vi "GUI.Config Pulse generator.vi"(8 "error in":errorcluster, 10 "Config HW":T2={"VISA Rigol DP832"="FA_Rigol_DP832", "Config Rigol DP832"=[], "CTA Test#"="", "FT_Handle"=0, "Espera acceso FT"=0, "VISA Tek MDO3104"="Osciloscopio_Tek_MDO3104", "VISA Key 81160A"="Generator_Key_81160A"} {"Config Rigol DP832"."Channel" items=["+30V Channel 1", "+30V Channel 2", "+5V Channel 3"]; "Config Rigol DP832"."V Limit" format="%.1g"; "Config Rigol DP832"."I Limit" format="%.1g"; "Config Rigol DP832"."V Out" format="%.1g"}, 11 "CONFIG GEN origen":T1[](array[typedef]) {"Vasic Theorical" min=1.0 max=1000000.0 step=1.0 format="%#_6pV"; "Frequency" min=0.001 max=333000000.0 step=1000.0 format="%#_6pHz"; "Leading Edge Time" min=1e-09 max=1.0 step=1e-10 format="%#_6ps"; "Trailing Edge Time" min=1e-09 max=1.0 step=1e-10 format="%#_6ps"; "Delay" min=0.0 max=1.0 step=1e-12 format="%#_6ps"; "Trigger Level Sync" items=["ECL", "TTL"]; "Trigger Sync Out" items=["AB"=3, "B"=2, "A"=1, "None"=0]; "Load" min=1.0 max=1000000.0 step=1.0 format="%#_6p"; "DC Offset" min=-10.0 max=10.0 step=0.1 format="%#_6pV"; "Amplitude" min=0.05 max=5.0 step=0.001 format="%#_6pV"; "Width Time" min=1.5e-09 max=1.0 step=1e-10 format="%#_6ps"; "Channel" items=["Channel1"=1, "Channel2"=2]}) -> (0 "error out":errorcluster={"status"=TRUE, "code"=-1073807346, "source"="Property Node (arg 1) in DP832_Write.vi->DP832_Enable ALL Output.vi->GUI.Config Pulse generator.vi"}, 3 "Array pulse Out":T1[](array[typedef])=[{"Channel"=1, "Frequency"=1000000.0, "Width Time"=3.3e-09, "Amplitude"=0.05, "DC Offset"=0.0, "Load"=500.0, "Leading Edge Time"=1e-09, "Trailing Edge Time"=1e-09, "Delay"=0.0, "Out"=TRUE, "/Out"=TRUE, "Trigger Level Sync"=1, "Trigger Sync Out"=1, "Vasic Theorical"=50.0}, {"Channel"=1, "Frequency"=1000000.0, "Width Time"=3.3e-09, "Amplitude"=0.1, "DC Offset"=0.0, "Load"=500.0, "Leading Edge Time"=1e-09, "Trailing Edge Time"=1e-09, "Delay"=0.0, "Out"=TRUE, "/Out"=TRUE, "Trigger Level Sync"=1, "Trigger Sync Out"=1, "Vasic Theorical"=50.0}, {"Channel"=1, "Frequency"=1000000.0, "Width Time"=3.3e-09, "Amplitude"=0.2, "DC Offset"=0.0, "Load"=500.0, "Leading Edge Time"=1e-09, "Trailing Edge Time"=1e-09, "Delay"=0.0, "Out"=TRUE, "/Out"=TRUE, "Trigger Level Sync"=1, "Trigger Sync Out"=1, "Vasic Theorical"=50.0}, {"Channel"=1, "Frequency"=1000000.0, "Width Time"=3.3e-09, "Amplitude"=0.3, "DC Offset"=0.0, "Load"=500.0, "Leading Edge Time"=1e-09, "Trailing Edge Time"=1e-09, "Delay"=0.0, "Out"=TRUE, "/Out"=TRUE, "Trigger Level Sync"=1, "Trigger Sync Out"=1, "Vasic Theorical"=50.0}, {"Channel"=1, "Frequency"=1000000.0, "Width Time"=3.3e-09, "Amplitude"=0.4, "DC Offset"=0.0, "Load"=500.0, "Leading Edge Time"=1e-09, "Trailing Edge Time"=1e-09, "Delay"=0.0, "Out"=TRUE, "/Out"=TRUE, "Trigger Level Sync"=1, "Trigger Sync Out"=1, "Vasic Theorical"=50.0}, {"Channel"=1, "Frequency"=1000000.0, "Width Time"=3.3e-09, "Amplitude"=0.5, "DC Offset"=0.0, "Load"=500.0, "Leading Edge Time"=1e-09, "Trailing Edge Time"=1e-09, "Delay"=0.0, "Out"=TRUE, "/Out"=TRUE, "Trigger Level Sync"=1, "Trigger Sync Out"=1, "Vasic Theorical"=50.0}, {"Channel"=1, "Frequency"=1000000.0, "Width Time"=3.3e-09, "Amplitude"=0.6, "DC Offset"=0.0, "Load"=500.0, "Leading Edge Time"=1e-09, "Trailing Edge Time"=1e-09, "Delay"=0.0, "Out"=TRUE, "/Out"=TRUE, "Trigger Level Sync"=1, "Trigger Sync Out"=1, "Vasic Theorical"=50.0}, {"Channel"=1, "Frequency"=1000000.0, "Width Time"=3.3e-09, "Amplitude"=0.7, "DC Offset"=0.0, "Load"=500.0, "Leading Edge Time"=1e-09, "Trailing Edge Time"=1e-09, "Delay"=0.0, "Out"=TRUE, "/Out"=TRUE, "Trigger Level Sync"=1, "Trigger Sync Out"=1, "Vasic Theorical"=50.0}, {"Channel"=1, "Frequency"=1000000.0, "Width Time"=3.3e-09, "Amplitude"=0.8, "DC Offset"=0.0, "Load"=500.0, "Leading Edge Time"=1e-09, "Trailing Edge Time"=1e-09, "Delay"=0.0, "Out"=TRUE, "/Out"=TRUE, "Trigger Level Sync"=1, "Trigger Sync Out"=1, "Vasic Theorical"=50.0}, {"Channel"=1, "Frequency"=1000000.0, "Width Time"=3.3e-09, "Amplitude"=0.9, "DC Offset"=0.0, "Load"=500.0, "Leading Edge Time"=1e-09, "Trailing Edge Time"=1e-09, "Delay"=0.0, "Out"=TRUE, "/Out"=TRUE, "Trigger Level Sync"=1, "Trigger Sync Out"=1, "Vasic Theorical"=50.0}, {"Channel"=1, "Frequency"=1000000.0, "Width Time"=3.3e-09, "Amplitude"=1.0, "DC Offset"=0.0, "Load"=500.0, "Leading Edge Time"=1e-09, "Trailing Edge Time"=1e-09, "Delay"=0.0, "Out"=TRUE, "/Out"=TRUE, "Trigger Level Sync"=1, "Trigger Sync Out"=1, "Vasic Theorical"=50.0}] {"Vasic Theorical" min=1.0 max=1000000.0 step=1.0 format="%#_6pV"; "Frequency" min=0.001 max=333000000.0 step=1000.0 format="%#_6pHz"; "Leading Edge Time" min=1e-09 max=1.0 step=1e-10 format="%#_6ps"; "Trailing Edge Time" min=1e-09 max=1.0 step=1e-10 format="%#_6ps"; "Delay" min=0.0 max=1.0 step=1e-12 format="%#_6ps"; "Trigger Level Sync" items=["ECL", "TTL"]; "Trigger Sync Out" items=["AB"=3, "B"=2, "A"=1, "None"=0]; "Load" min=1.0 max=1000000.0 step=1.0 format="%#_6p"; "DC Offset" min=-10.0 max=10.0 step=0.1 format="%#_6pV"; "Amplitude" min=0.05 max=5.0 step=0.001 format="%#_6pV"; "Width Time" min=1.5e-09 max=1.0 step=1e-10 format="%#_6ps"; "Channel" items=["Channel1"=1, "Channel2"=2]})   [LabVIEW 2019]
uses:
  Machine State generador pulsos.ctl
  GenPulse_configurar.ctl
  Rigol DP832/DP832_Control Channels.ctl
  TEST.TEST CONFIG HW.ctl
  Test_Conjunto Folder/Rigol DP832/DP832_Control Behavior.ctl
  Viejos/Alfredo LABVIEW/Set-up verificador ASICs/Lib Agilent 81160A/Agilent 81150/Agilent 81150.lvlib
  Tektronix DPO MSO 2000 4000 Series/Tektronix DPO MSO 2000 4000 Series.lvlib
  RIGOL DP1000 Series/RIGOL DP1000 Series.lvlib
panel:
  out "Values Generator":T1[](array[typedef]) {"Vasic Theorical" min=1.0 max=1000000.0 step=1.0 format="%#_6pV"; "Frequency" min=0.001 max=333000000.0 step=1000.0 format="%#_6pHz"; "Leading Edge Time" min=1e-09 max=1.0 step=1e-10 format="%#_6ps"; "Trailing Edge Time" min=1e-09 max=1.0 step=1e-10 format="%#_6ps"; "Delay" min=0.0 max=1.0 step=1e-12 format="%#_6ps"; "Trigger Level Sync" items=["ECL", "TTL"]; "Trigger Sync Out" items=["AB"=3, "B"=2, "A"=1, "None"=0]; "Load" min=1.0 max=1000000.0 step=1.0 format="%#_6p"; "DC Offset" min=-10.0 max=10.0 step=0.1 format="%#_6pV"; "Amplitude" min=0.05 max=5.0 step=0.001 format="%#_6pV"; "Width Time" min=1.5e-09 max=1.0 step=1e-10 format="%#_6ps"; "Channel" items=["Channel1"=1, "Channel2"=2]}
  out "VISA Tek MDO3104":refnum<visa-resource-name>
  out "VISA Generator Key 81160A":refnum<visa-resource-name>
  out "Config Rigol DP832":T4(array[cluster]) {"Channel" items=["+30V Channel 1", "+30V Channel 2", "+5V Channel 3"]; "V Limit" min=0.0 max=6.0 step=0.1 format="%.1g"; "I Limit" min=0.0 max=1.0 step=0.1 format="%.1g"; "V Out" min=0.0 max=6.0 step=0.01 format="%.2g"}
  out "VISA Rigol DP832":refnum<visa-resource-name>
  in  "Enum info":T5
  in  "visualize":enum32{"Page 1", "Page 2"}(tab)
  in  "Set Default":bool
  in  "VIn ASIC":u16(ring) items=["50 mV", "100 mV", "200 mV", "300 mV", "400 mV", "500 mV", "600 mV", "700 mV", "800 mV", "900 mV", "1000 mV"]
  in  "Save":bool
  in  "Quit":bool
  in  "Test":bool=TRUE
  in  "CONFIG GEN":T1[](array[typedef])=[{"Channel"=1, "Frequency"=1000000.0, "Width Time"=3.3e-09, "Amplitude"=0.05, "DC Offset"=0.0, "Load"=500.0, "Leading Edge Time"=1e-09, "Trailing Edge Time"=1e-09, "Delay"=0.0, "Out"=TRUE, "/Out"=TRUE, "Trigger Level Sync"=1, "Trigger Sync Out"=1, "Vasic Theorical"=50.0}, {"Channel"=1, "Frequency"=1000000.0, "Width Time"=3.3e-09, "Amplitude"=0.1, "DC Offset"=0.0, "Load"=500.0, "Leading Edge Time"=1e-09, "Trailing Edge Time"=1e-09, "Delay"=0.0, "Out"=TRUE, "/Out"=TRUE, "Trigger Level Sync"=1, "Trigger Sync Out"=1, "Vasic Theorical"=50.0}, {"Channel"=1, "Frequency"=1000000.0, "Width Time"=3.3e-09, "Amplitude"=0.2, "DC Offset"=0.0, "Load"=500.0, "Leading Edge Time"=1e-09, "Trailing Edge Time"=1e-09, "Delay"=0.0, "Out"=TRUE, "/Out"=TRUE, "Trigger Level Sync"=1, "Trigger Sync Out"=1, "Vasic Theorical"=50.0}, {"Channel"=1, "Frequency"=1000000.0, "Width Time"=3.3e-09, "Amplitude"=0.3, "DC Offset"=0.0, "Load"=500.0, "Leading Edge Time"=1e-09, "Trailing Edge Time"=1e-09, "Delay"=0.0, "Out"=TRUE, "/Out"=TRUE, "Trigger Level Sync"=1, "Trigger Sync Out"=1, "Vasic Theorical"=50.0}, {"Channel"=1, "Frequency"=1000000.0, "Width Time"=3.3e-09, "Amplitude"=0.4, "DC Offset"=0.0, "Load"=500.0, "Leading Edge Time"=1e-09, "Trailing Edge Time"=1e-09, "Delay"=0.0, "Out"=TRUE, "/Out"=TRUE, "Trigger Level Sync"=1, "Trigger Sync Out"=1, "Vasic Theorical"=50.0}, {"Channel"=1, "Frequency"=1000000.0, "Width Time"=3.3e-09, "Amplitude"=0.5, "DC Offset"=0.0, "Load"=500.0, "Leading Edge Time"=1e-09, "Trailing Edge Time"=1e-09, "Delay"=0.0, "Out"=TRUE, "/Out"=TRUE, "Trigger Level Sync"=1, "Trigger Sync Out"=1, "Vasic Theorical"=50.0}, {"Channel"=1, "Frequency"=1000000.0, "Width Time"=3.3e-09, "Amplitude"=0.6, "DC Offset"=0.0, "Load"=500.0, "Leading Edge Time"=1e-09, "Trailing Edge Time"=1e-09, "Delay"=0.0, "Out"=TRUE, "/Out"=TRUE, "Trigger Level Sync"=1, "Trigger Sync Out"=1, "Vasic Theorical"=50.0}, {"Channel"=1, "Frequency"=1000000.0, "Width Time"=3.3e-09, "Amplitude"=0.7, "DC Offset"=0.0, "Load"=500.0, "Leading Edge Time"=1e-09, "Trailing Edge Time"=1e-09, "Delay"=0.0, "Out"=TRUE, "/Out"=TRUE, "Trigger Level Sync"=1, "Trigger Sync Out"=1, "Vasic Theorical"=50.0}, {"Channel"=1, "Frequency"=1000000.0, "Width Time"=3.3e-09, "Amplitude"=0.8, "DC Offset"=0.0, "Load"=500.0, "Leading Edge Time"=1e-09, "Trailing Edge Time"=1e-09, "Delay"=0.0, "Out"=TRUE, "/Out"=TRUE, "Trigger Level Sync"=1, "Trigger Sync Out"=1, "Vasic Theorical"=50.0}, {"Channel"=1, "Frequency"=1000000.0, "Width Time"=3.3e-09, "Amplitude"=0.9, "DC Offset"=0.0, "Load"=500.0, "Leading Edge Time"=1e-09, "Trailing Edge Time"=1e-09, "Delay"=0.0, "Out"=TRUE, "/Out"=TRUE, "Trigger Level Sync"=1, "Trigger Sync Out"=1, "Vasic Theorical"=50.0}, {"Channel"=1, "Frequency"=1000000.0, "Width Time"=3.3e-09, "Amplitude"=1.0, "DC Offset"=0.0, "Load"=500.0, "Leading Edge Time"=1e-09, "Trailing Edge Time"=1e-09, "Delay"=0.0, "Out"=TRUE, "/Out"=TRUE, "Trigger Level Sync"=1, "Trigger Sync Out"=1, "Vasic Theorical"=50.0}] {"Vasic Theorical" min=1.0 max=1000000.0 step=1.0 format="%#_6pV"; "Frequency" min=0.001 max=333000000.0 step=1000.0 format="%#_6pHz"; "Leading Edge Time" min=1e-09 max=1.0 step=1e-10 format="%#_6ps"; "Trailing Edge Time" min=1e-09 max=1.0 step=1e-10 format="%#_6ps"; "Delay" min=0.0 max=1.0 step=1e-12 format="%#_6ps"; "Trigger Level Sync" items=["ECL", "TTL"]; "Trigger Sync Out" items=["AB"=3, "B"=2, "A"=1, "None"=0]; "Load" min=1.0 max=1000000.0 step=1.0 format="%#_6p"; "DC Offset" min=-10.0 max=10.0 step=0.1 format="%#_6pV"; "Amplitude" min=0.05 max=5.0 step=0.001 format="%#_6pV"; "Width Time" min=1.5e-09 max=1.0 step=1e-10 format="%#_6ps"; "Channel" items=["Channel1"=1, "Channel2"=2]}
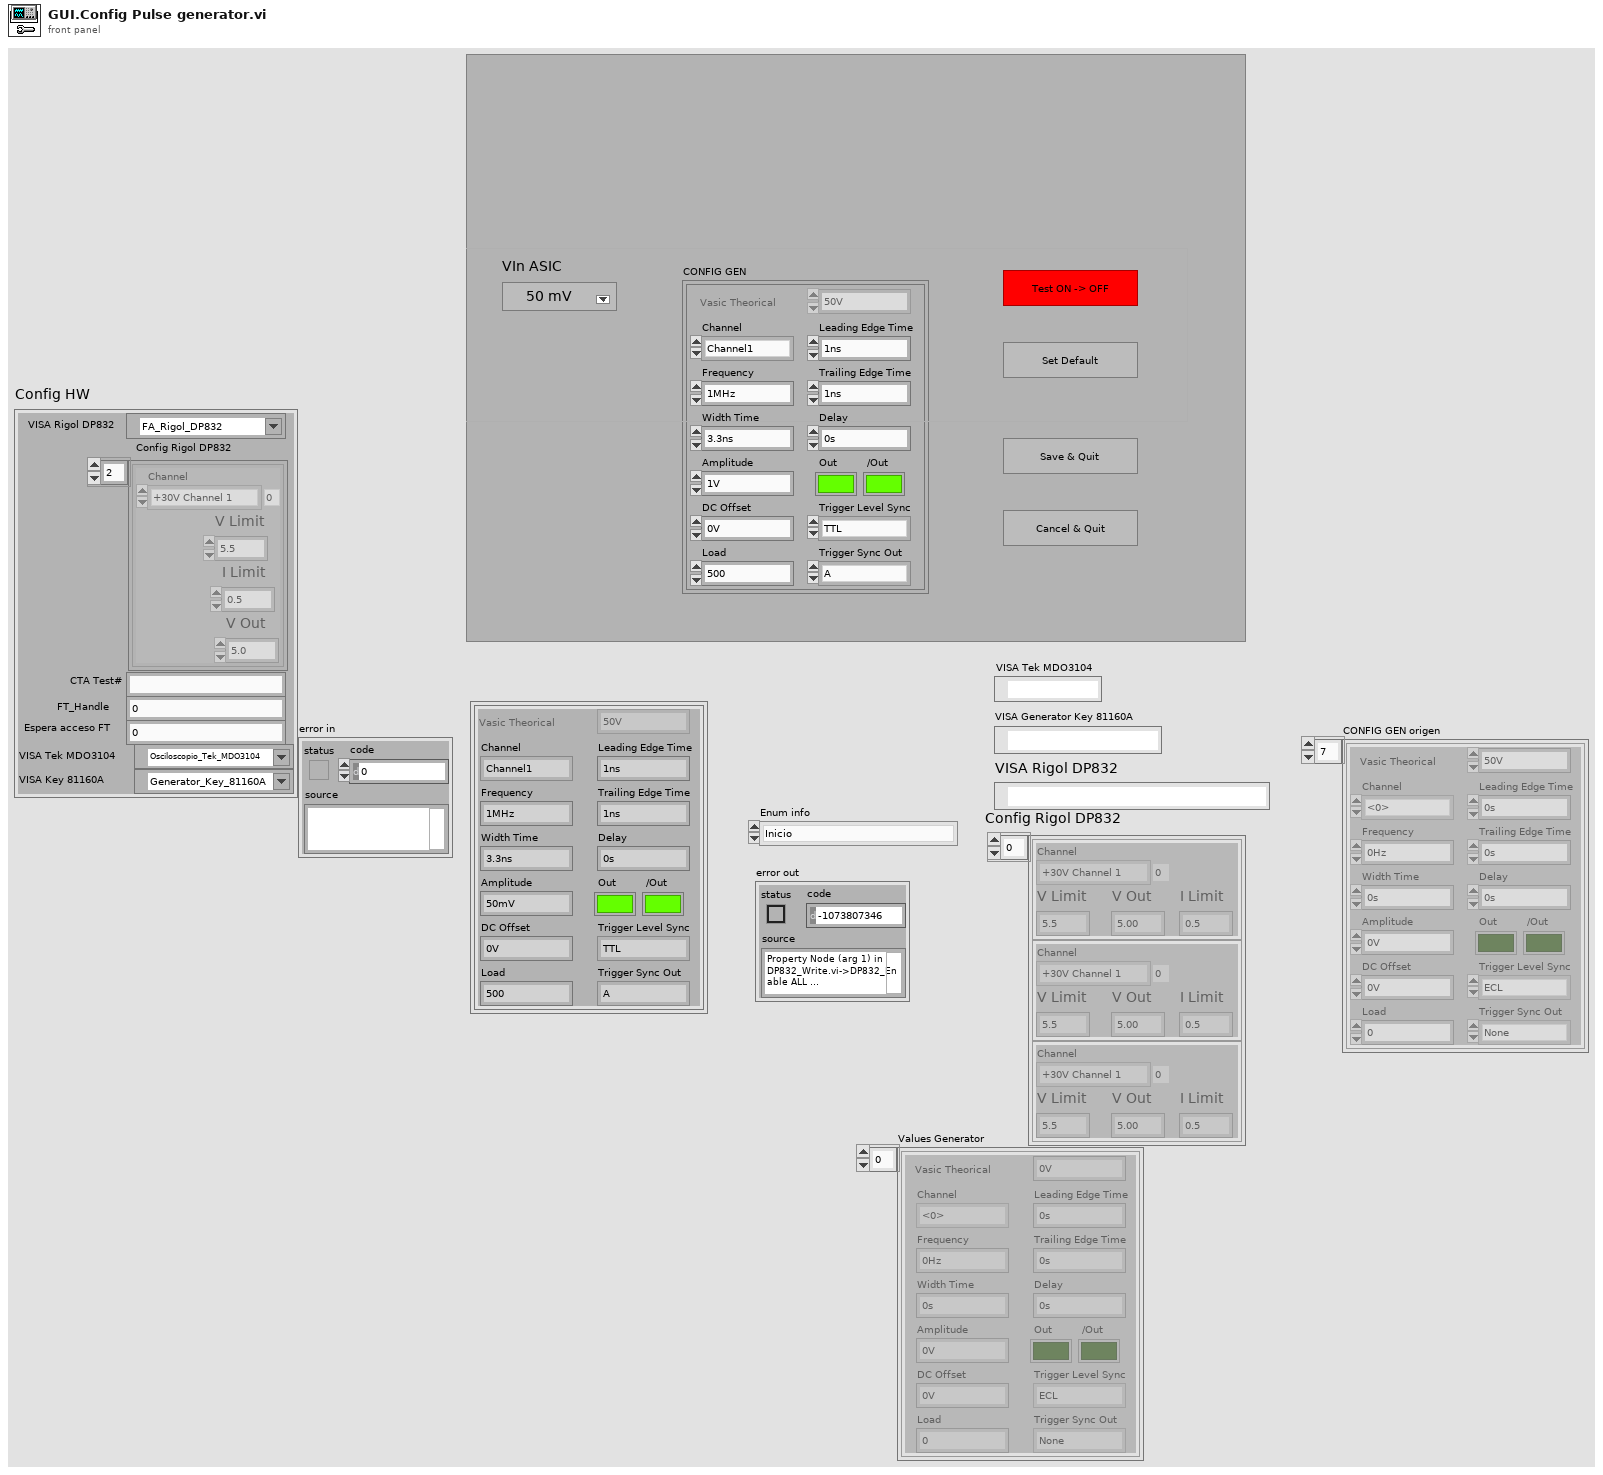
[diagram p1: front panel]
types:
  T1 = typedef "GenPulse_configurar.ctl" = cluster{"Channel":u16, "Frequency":dbl, "Width Time":dbl, "Amplitude":dbl, "DC Offset":dbl, "Load":dbl, "Leading Edge Time":dbl, "Trailing Edge Time":dbl, "Delay":dbl, "Out":bool, "/Out":bool, "Trigger Level Sync":u16, "Trigger Sync Out":u16, "Vasic Theorical":dbl}
  T2 = typedef "TEST.TEST CONFIG HW.ctl" = cluster{"VISA Rigol DP832":refnum<visa-resource-name>, "Config Rigol DP832":cluster{"Channel":T3, "V Limit":dbl, "I Limit":dbl, "V Out":dbl}[], "CTA Test#":string, "FT_Handle":u32, "Espera acceso FT":u32, "VISA Tek MDO3104":refnum<visa-resource-name>, "VISA Key 81160A":refnum<visa-resource-name>}
  T3 = typedef "DP832_Control Channels.ctl" = i32
  T4 = cluster{"Channel":T3, "V Limit":dbl, "I Limit":dbl, "V Out":dbl}[]
  T5 = typedef "Machine State generador pulsos.ctl" = enum16{"Inicio", "Inicia HW", "Idle", "Test On", "Test Off", "Set default", "Cambio pulso", "Error Labview", "Error maquina", "Cierra HW", "No salvar", "Fin", "Bye"}
  T6 = typedef "DP832_Control Behavior.ctl" = u16
  T7 = enum16{"Left Button", "Center Button", "Right Button", "Window Close"}
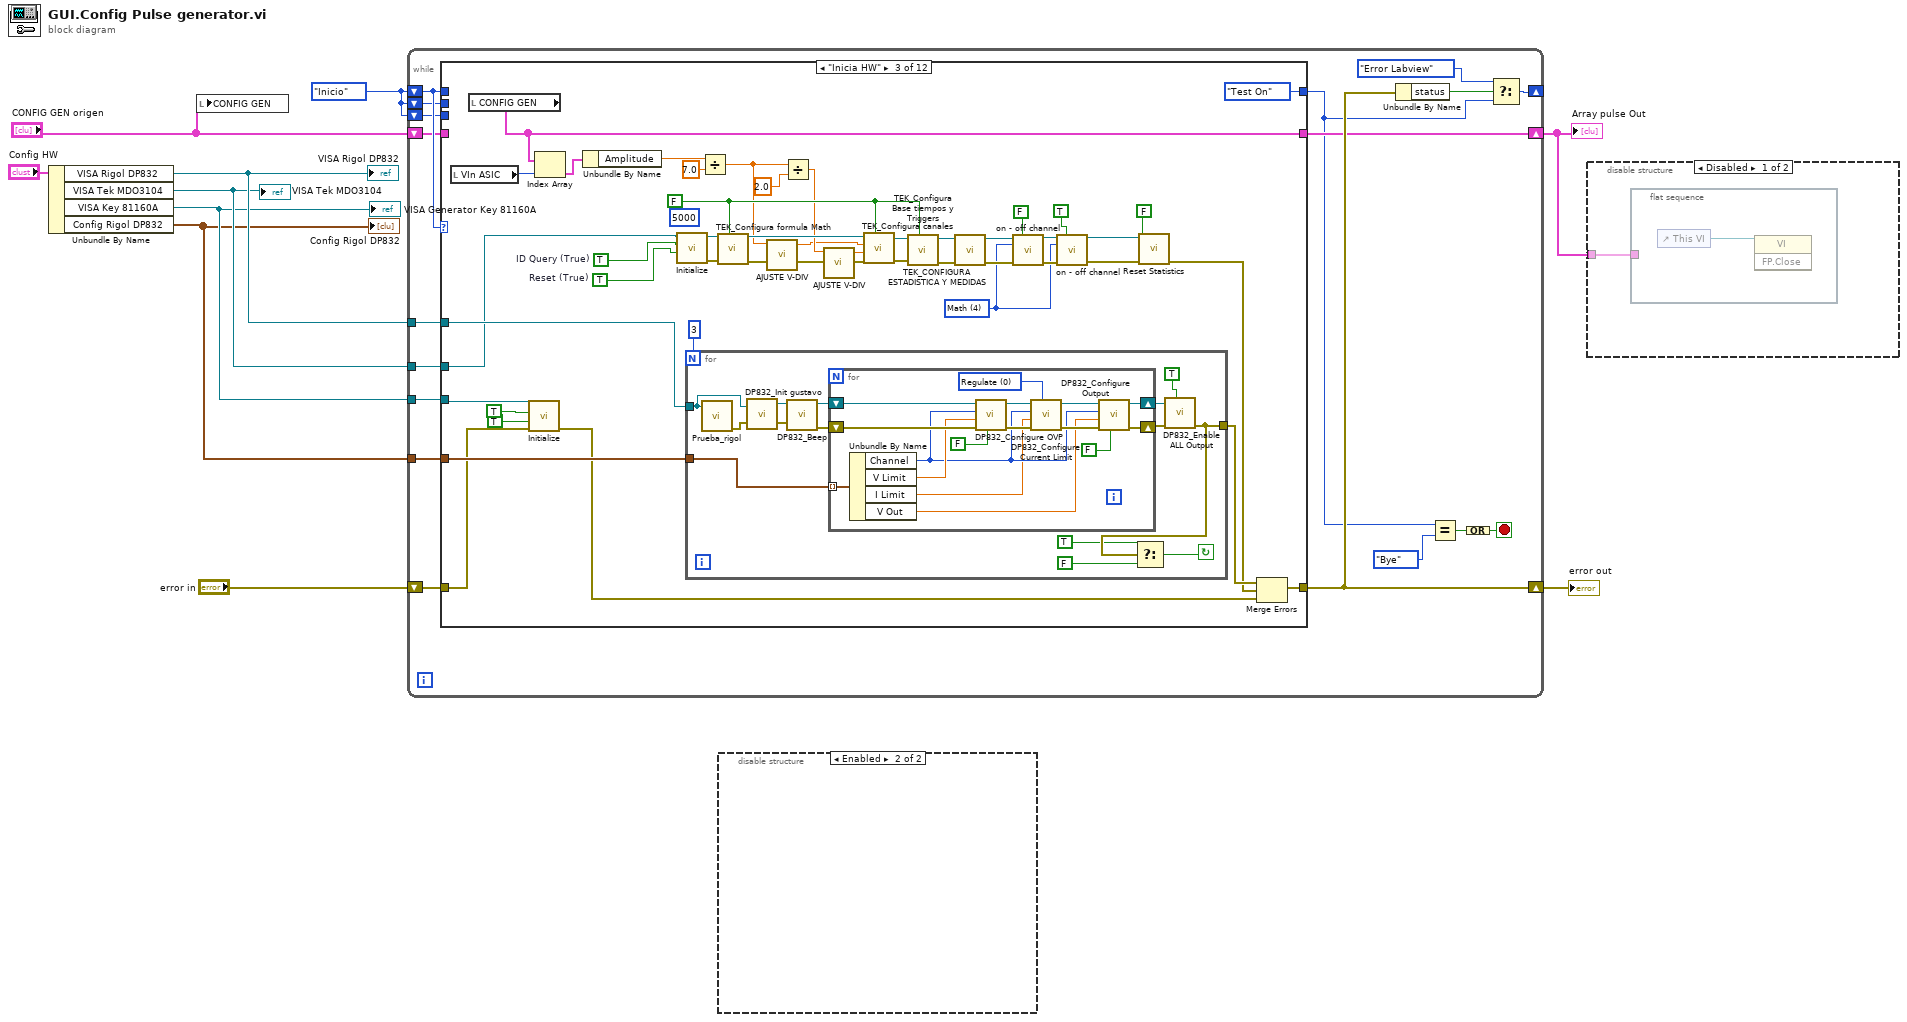
[diagram p0: block diagram]
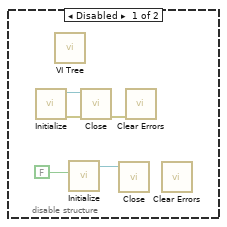
[diagram p3: hidden frame]
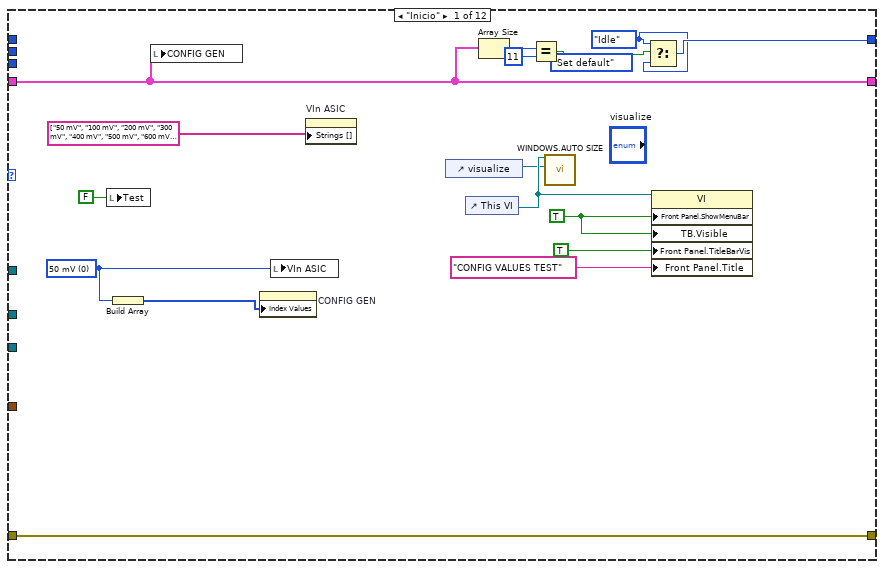
[diagram p4: hidden frame]
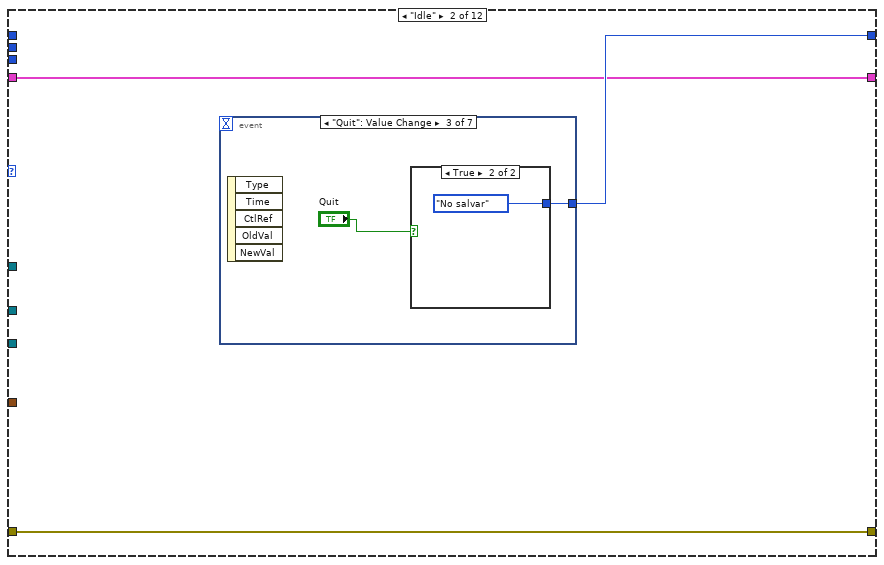
[diagram p5: hidden frame]
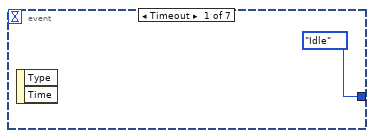
[diagram p6: hidden frame]
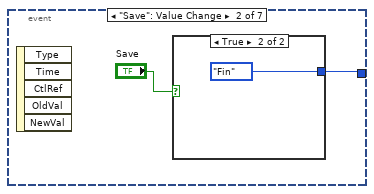
[diagram p7: hidden frame]
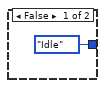
[diagram p8: hidden frame]
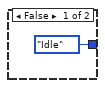
[diagram p9: hidden frame]
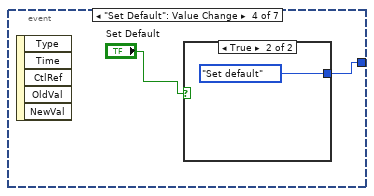
[diagram p10: hidden frame]
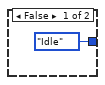
[diagram p11: hidden frame]
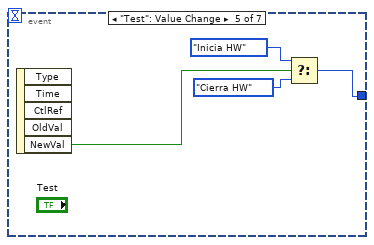
[diagram p12: hidden frame]
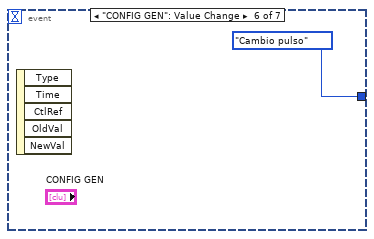
[diagram p13: hidden frame]
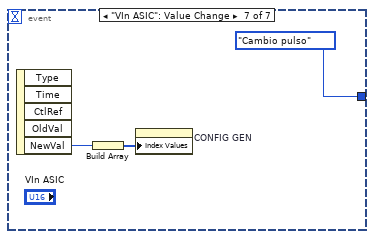
[diagram p14: hidden frame]
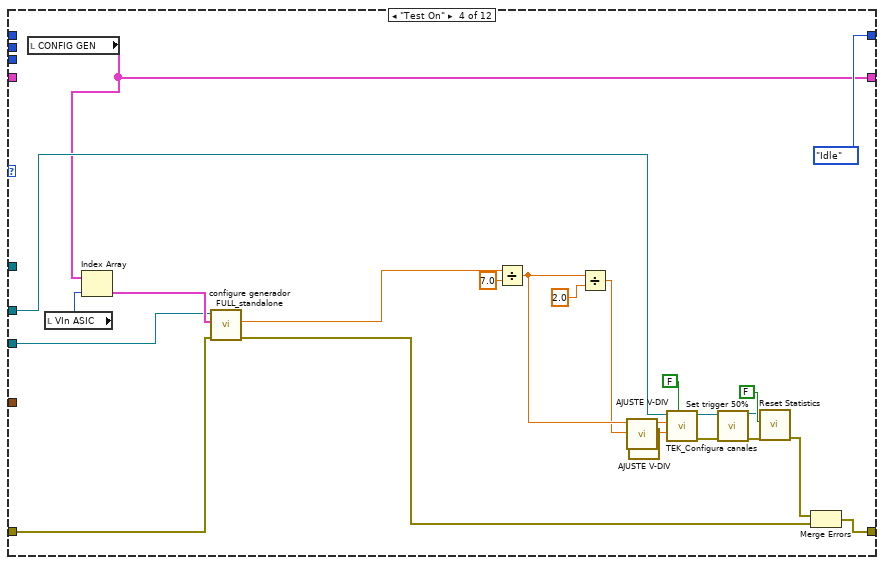
[diagram p15: hidden frame]
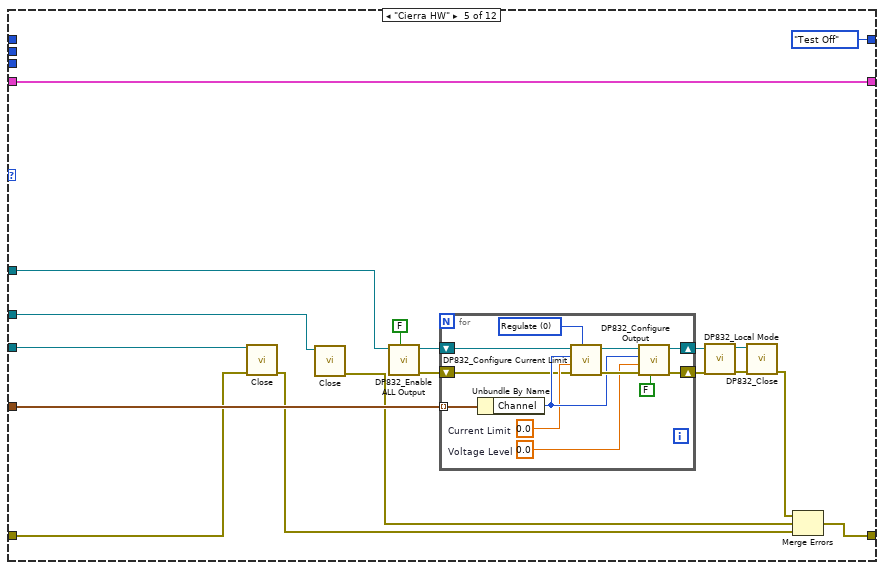
[diagram p16: hidden frame]
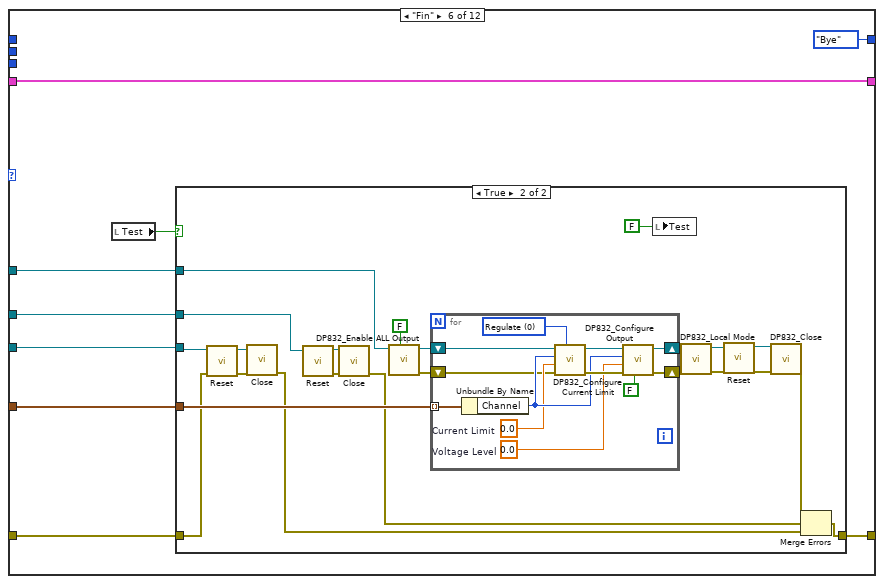
[diagram p17: hidden frame]
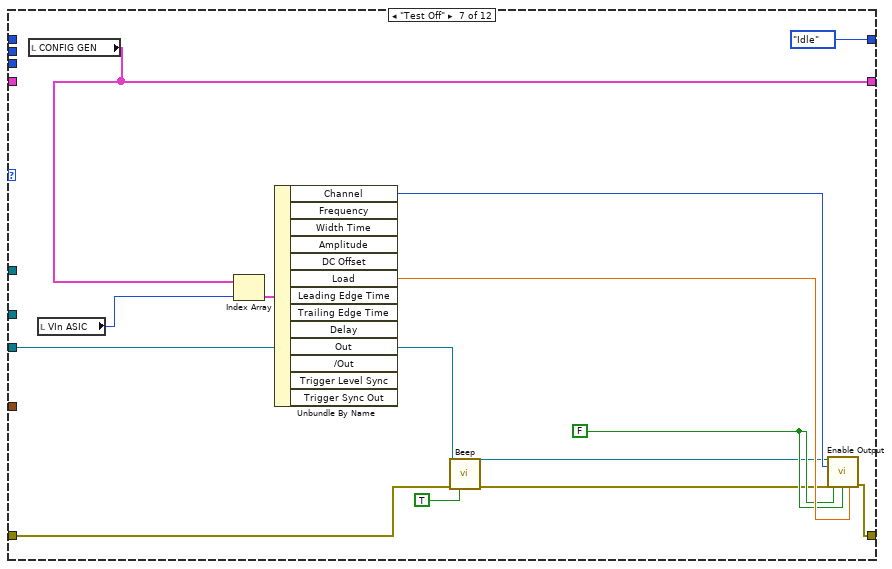
[diagram p19: hidden frame]
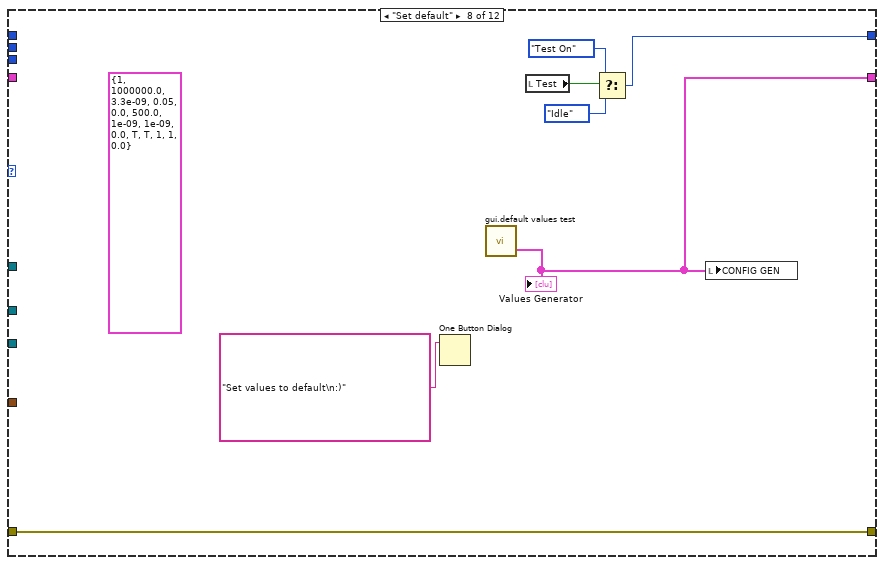
[diagram p20: hidden frame]
diagram:
  w8 = Machine_State_generador_pulsos."Inicio" ("Enum")
  n1 = Unbundle By Name("Config HW") -> ("VISA Rigol DP832"=w6:refnum<visa-resource-name>, "VISA Tek MDO3104"=w5:refnum<visa-resource-name>, "VISA Key 81160A"=w4:refnum<visa-resource-name>, "Config Rigol DP832"=w3:T4)
  "VISA Generator Key 81160A" <- w4
  "VISA Rigol DP832" <- w6
  "Config Rigol DP832" <- w3
  "VISA Tek MDO3104" <- w5
  n2 = local write "CONFIG GEN"("CONFIG GEN origen") -> ()
  n3 = while {
    shift-right: [w20] -> _
    shift-left: w8 -> [w28]
    tunnel: w4 -> [w26]
    shift-right: [w24] -> w9
    shift-left: "error in" -> [w25]
    shift-right: [w19] -> w2
    shift-left: "CONFIG GEN origen" -> [w18]
    shift-left: w8 -> [w17]
    shift-left: w8 -> [w16]
    tunnel: w3 -> [w13]
    tunnel: w6 -> [w12]
    tunnel: w5 -> [w11]
    stop <- w22 stop-if-true
    n4 = case shown="\"Inicia HW\"" w28 {
      tunnel: [w31 w47 Machine_State_generador_pulsos."Test On" ("Enum") Machine_State_generador_pulsos."Idle" ("Enum") Machine_State_generador_pulsos."Test Off" ("Enum") Machine_State_generador_pulsos."Bye" ("Enum") Machine_State_generador_pulsos."Idle" ("Enum") w256 w262 w272 w309 Machine_State_generador_pulsos."Fin" ("y")] -> w14
      tunnel: w28 -> [_ _ _ _ _ _ _ _ _ _ w307 _]
      tunnel: w26 -> [_ _ w106 w161 w181 w203 w246 _ _ w270 _ _]
      tunnel: [w37 w46 w104 w159 w177 w199 w249 w260 w266 w269 w316 w319] -> w24
      tunnel: w25 -> [w37 w46 w105 w162 w178 w200 w244 w260 w266 w283 w316 w319]
      tunnel: w18 -> [w35 w45 _ _ w183 w196 _ _ _ w284 w315 _]
      tunnel: [w35 w45 w74 w143 w183 w196 w241 w255 w261 w284 w315 w317] -> w19
      tunnel: w17 -> [_ _ _ _ _ _ _ _ _ w273 w306 _]
      tunnel: w16 -> [_ _ _ _ _ _ _ _ _ _ w305 _]
      tunnel: w13 -> [_ _ w112 _ w182 w204 _ _ _ _ _ _]
      tunnel: w12 -> [_ _ w111 _ w179 w201 _ _ _ w268 _ _]
      tunnel: w11 -> [_ _ w71 w153 w180 w202 _ _ _ w267 _ _]
      frame "Inicio" {
        (unwired) Machine_State_generador_pulsos."Set default" ("f")
        w39 = TRUE ("Front Panel Window:Show Menu Bar")
        w43 = u16 0 items=["50 mV", "100 mV", "200 mV", "300 mV", "400 mV", "500 mV", "600 mV", "700 mV", "800 mV", "900 mV", "1000 mV"] ("Vin test Asic")
        w29 = Machine_State_generador_pulsos."Idle" ("Enum")
        n5 = local write "Test"(FALSE ("Test")) -> ()
        n6 = Build Array(w43) -> (w36:u16[])
        n7 = local write "CONFIG GEN"(w35) -> ()
        n8 = property on="CONFIG GEN" class="Arr (strict)"("Index Values"=w36) -> ()  [unwired: 2 in, 2 out]
        n9 = local write "VIn ASIC"(w43) -> ()
        n10 = property on="VIn ASIC" class="Ring (strict)"("Strings []"=string[] ["50 mV", "100 mV", "200 mV", "300 mV", "400 mV", "500 mV", "600 mV", "700 mV", "800 mV", "900 mV", "1000 mV"] ("Column Headers")) -> ()  [unwired: 2 in, 2 out]
        n11 = control-ref of="visualize"() -> (w38:refnum<vi>)
        n12 = control-ref of="This VI"() -> (w42:refnum<vi>)
        n13 = Array Size(array=w35) -> (size(s)=w34:i32)
        n14 = Equal?(x=w34, y=11) -> (x = y?=w32:bool)
        n15 = call "WINDOWS.AUTO SIZE.vi"("TAB.AutoAjuste"=w38, "This VI"=w42) -> ()  [unwired: 5 in, 1 out]
        n16 = Select(t=w29, s=w32, f=w29) -> (s? t:f=w31:T5)
        n17 = property class="VI"(reference=w42, "Front Panel.ShowMenuBar"=w39, "TB.Visible"=w39, "Front Panel.TitleBarVis"=TRUE ("Front Panel Window:Title Bar Visible"), "Front Panel.Title"="CONFIG VALUES TEST" ("Front Panel Window:Title")) -> ()  [unwired: 1 in, 2 out]
      }
      frame "Idle" {
        n18 = event shown="[2] \"Quit\": Value Change" {
          selector: _ -> [_ _ _ _ _ _ _]
          dyn-events: _ -> [_ _ _ _ _ _ _]
          timeout: _ -> [_ _ _ _ _ _ _]
          tunnel: [Machine_State_generador_pulsos."Idle" ("Enum") w50 w54 w58 w61 Machine_State_generador_pulsos."Cambio pulso" ("Enum") Machine_State_generador_pulsos."Cambio pulso" ("Enum")] -> w47
          event Timeout {
            n19 = event-data() -> ()  [unwired: 1 in, 2 out]
          }
          event "Save": Value Change {
            n20 = event-data() -> ()  [unwired: 1 in, 5 out]
            n21 = case shown="True" "Save" {
              tunnel: [Machine_State_generador_pulsos."Idle" ("Enum") Machine_State_generador_pulsos."Fin" ("Enum")] -> w50
              frame False {
              }
              frame True {
              }
            }
          }
          event "Quit": Value Change {
            n22 = event-data() -> ()  [unwired: 1 in, 5 out]
            n23 = case shown="True" "Quit" {
              tunnel: [Machine_State_generador_pulsos."Idle" ("Enum") Machine_State_generador_pulsos."No salvar" ("Enum")] -> w54
              frame False {
              }
              frame True {
              }
            }
          }
          event "Set Default": Value Change {
            n24 = event-data() -> ()  [unwired: 1 in, 5 out]
            n25 = case shown="True" "Set Default" {
              tunnel: [Machine_State_generador_pulsos."Idle" ("Enum") Machine_State_generador_pulsos."Set default" ("Enum")] -> w58
              frame False {
              }
              frame True {
              }
            }
          }
          event "Test": Value Change {
            n26 = event-data() -> ("NewVal"=w62:bool)  [unwired: 1 in, 4 out]
            n27 = Select(t=Machine_State_generador_pulsos."Inicia HW" ("Enum"), s=w62, f=Machine_State_generador_pulsos."Cierra HW" ("Enum")) -> (s? t:f=w61:T5)
          }
          event "CONFIG GEN": Value Change {
            n28 = event-data() -> ()  [unwired: 1 in, 5 out]
          }
          event "VIn ASIC": Value Change {
            n29 = event-data() -> ("NewVal"=w68:u16)  [unwired: 1 in, 4 out]
            n30 = Build Array(w68) -> (w66:u16[])
            n31 = property on="CONFIG GEN" class="Arr (strict)"("Index Values"=w66) -> ()  [unwired: 2 in, 2 out]
          }
        }
      }
      frame "Inicia HW" {
        w92 = FALSE ("Debug")
        w96 = u16 4 items=["Channel 1", "Channel 2", "Channel 3", "Channel 4", "Math", "Reference 1", "Reference 2", "Reference 3", "Reference 4", "Bus 1", "Bus 2"] ("Channel (0: Channel 1)")
        (unwired) u32 5000 ("VISA Open timeout (0)")
        w69 = TRUE  # Reset (True)
        w70 = TRUE  # ID Query (True)
        n32 = local read "VIn ASIC"() -> (w91:u16)
        n33 = local read "CONFIG GEN"() -> (w74:T1[])
        n34 = call <instrlib>:"Initialize.vi"("error in (no error)"=w105, "Reset (True)"=TRUE, "ID Query (True)"=TRUE, "VISA resource name"=w106) -> ("error out"=w102:errorcluster)  [unwired: 6 in, 1 out]
        n35 = Index Array(array=w74, index=w91) -> (element=w90:T1)
        n36 = Unbundle By Name(w90) -> ("Amplitude"=w88:dbl)
        n37 = call <instrlib>:"Initialize.vi"("Reset (True)"=w69, "ID Query (True)"=w70, "VISA resource name"=w71) -> ("error out"=w73:errorcluster, "VISA resource name out"=w72:refnum<visa-resource-name>)  [unwired: 7 in]
        n38 = for {
          N: 3 -> [_]
          tunnel: [w118] -> w103
          tunnel: w112 -> [w121]
          tunnel: w111 -> [w113]
          stop <- w116 continue-if-true
          n39 = call "Prueba_rigol.vi"("VISA IN"=w113) -> ("error out 2"=w114:errorcluster)  [unwired: 9 in, 1 out]
          n40 = call "DP832_Init gustavo.vi"("error in (no error)"=w114, "VISA resource name 2"=w113) -> ("error out"=w119:errorcluster, "VISA resource name"=w120:refnum<visa-resource-name>)
          n41 = call "DP832_Beep.vi"("error in (no error)"=w119, "VISA resource name"=w120) -> ("error out"=w125:errorcluster, "VISA resource name out"=w126:refnum<visa-resource-name>)  [unwired: 8 in]
          n42 = for {
            shift-right: [w132] -> w123
            shift-left: w125 -> [w134]
            shift-right: [w133] -> w124
            shift-left: w126 -> [w135]
            tunnel: w121 -> [w131] mode=indexing
            w136 = T6 0 items=["Regulate", "Trip"] ("Behavior (0: Regulate)")
            n43 = Unbundle By Name(w131) -> ("Channel"=w129:T3, "V Limit"=w130:dbl, "I Limit"=w128:dbl, "V Out"=w127:dbl)
            n44 = call "DP832_Configure OVP.vi"("Enable OVP (T: Enable)"=FALSE, "error in (no error)"=w134, "Voltage Limit"=w130, "Channel"=w129, "VISA resource name"=w135) -> ("error out"=w139:errorcluster, "VISA resource name out"=w138:refnum<visa-resource-name>)  [unwired: 5 in]
            n45 = call "DP832_Configure Current Limit.vi"("Behavior"=w136, "error in (no error)"=w139, "Current Limit"=w128, "Channel"=w129, "VISA resource name"=w138) -> ("error out"=w141:errorcluster, "VISA resource name out"=w142:refnum<visa-resource-name>)  [unwired: 5 in]
            n46 = call "DP832_Configure Output.vi"("Enable Output (T: Enable)"=FALSE, "error in (no error)"=w141, "Voltage Level"=w127, "Channel"=w129, "VISA resource name"=w142) -> ("error out"=w132:errorcluster, "VISA resource name out"=w133:refnum<visa-resource-name>)  [unwired: 5 in]
          }
          n47 = call "DP832_Enable ALL Output.vi"("Enable Output (T: Enable)"=TRUE, "error in (no error)"=w123, "VISA resource name"=w124) -> ("error out"=w118:errorcluster)  [unwired: 7 in, 1 out]
          n48 = Select(t=TRUE, s=w118, f=FALSE) -> (s? t:f=w116:bool)
        }
        n49 = Divide(x=w88, y=7.0) -> (x/y=w78:dbl)
        n50 = call "TEK_Configura formula Math.vi"("Debug"=w92, "error out"=w73, "VISA resource name out 2"=w72) -> ("error out 2"=w81:errorcluster, "VISA resource name out"=w82:refnum<visa-resource-name>)  [unwired: 7 in]
        n51 = call "AJUSTE V-DIV.vi"("y 2"=w78) -> ("y"=w75:dbl)  [unwired: 10 in]
        n52 = Divide(x=w78, y=2.0) -> (x/y=w77:dbl)
        n53 = call "AJUSTE V-DIV.vi"("y 2"=w77) -> ("y"=w76:dbl)  [unwired: 10 in]
        n54 = call "TEK_Configura canales.vi"("Debug"=w92, "error out 2"=w81, "ch2 ch3 V/Div"=w76, "Math V/Div"=w75, "VISA resource name out"=w82) -> ("error out"=w86:errorcluster, "VISA resource name out 2"=w83:refnum<visa-resource-name>)  [unwired: 5 in]
        n55 = call "TEK_Configura Base tiempos y Triggers.vi"("Debug"=w92, "error out 2"=w86, "VISA resource name out 2"=w83) -> ("error out"=w85:errorcluster, "VISA resource name out"=w84:refnum<visa-resource-name>)  [unwired: 7 in]
        n56 = call "TEK_CONFIGURA ESTADISTICA Y MEDIDAS.vi"("error out"=w85, "VISA resource name out"=w84) -> ("error out 2"=w101:errorcluster, "VISA resource name out 2"=w99:refnum<visa-resource-name>)  [unwired: 8 in]
        n57 = call "on - off channel.vi"("VISA resource name"=w99, "Enable Channel (T: Enable)"=FALSE, "Channel (0: Channel 1)"=w96, "error in (no error)"=w101) -> ("VISA resource name out"=w98:refnum<visa-resource-name>, "error out"=w100:errorcluster)  [unwired: 10 in]
        n58 = call "on - off channel.vi"("VISA resource name"=w98, "Enable Channel (T: Enable)"=TRUE, "Channel (0: Channel 1)"=w96, "error in (no error)"=w100) -> ("VISA resource name out"=w80:refnum<visa-resource-name>, "error out"=w79:errorcluster)  [unwired: 10 in]
        n59 = call "Reset Statistics.vi"("error in (no error)"=w79, "Wait medida"=FALSE, "VISA resource name"=w80) -> ("error out"=w93:errorcluster)  [unwired: 7 in, 1 out]
        n60 = Merge Errors(w103, w93, w102) -> (w104:errorcluster)
      }
      frame "Test On" {
        n61 = local read "CONFIG GEN"() -> (w143:T1[])
        n62 = local read "VIn ASIC"() -> (w165:u16)
        n63 = Index Array(array=w143, index=w165) -> (element=w164:T1)
        n64 = call "configure generador FULL_standalone.vi"("error in"=w162, "Config Pulse"=w164, "VISA Key 81160A"=w161) -> ("error out"=w144:errorcluster, "Amplitude"=w150:dbl)  [unwired: 6 in, 1 out]
        n65 = Divide(x=w150, y=7.0) -> (x/y=w146:dbl)
        n66 = Divide(x=w146, y=2.0) -> (x/y=w145:dbl)
        n67 = call "AJUSTE V-DIV.vi"("y 2"=w146) -> ("y"=w147:dbl)  [unwired: 10 in]
        n68 = call "AJUSTE V-DIV.vi"("y 2"=w145) -> ("y"=w148:dbl)  [unwired: 10 in]
        n69 = call "TEK_Configura canales.vi"("Debug"=FALSE, "ch2 ch3 V/Div"=w148, "Math V/Div"=w147, "VISA resource name out"=w153) -> ("error out"=w155:errorcluster, "VISA resource name out 2"=w154:refnum<visa-resource-name>)  [unwired: 6 in]
        n70 = call "Set trigger 50%.vi"("error in (no error)"=w155, "VISA resource name"=w154) -> ("error out"=w156:errorcluster, "VISA resource name out"=w157:refnum<visa-resource-name>)  [unwired: 8 in]
        n71 = call "Reset Statistics.vi"("error in (no error)"=w156, "Wait medida"=FALSE, "VISA resource name"=w157) -> ("error out"=w158:errorcluster)  [unwired: 7 in, 1 out]
        n72 = Merge Errors(w158, w144) -> (w159:errorcluster)
      }
      frame "Cierra HW" {
        n73 = call <instrlib>:"Close.vi"("error in (no error)"=w178, "VISA resource name"=w181) -> ("error out"=w166:errorcluster)  [unwired: 9 in]
        n74 = call <instrlib>:"Close.vi"("VISA resource name"=w180) -> ("error out"=w167:errorcluster)  [unwired: 10 in]
        n75 = call "DP832_Enable ALL Output.vi"("Enable Output (T: Enable)"=FALSE, "VISA resource name"=w179) -> ("error out"=w173:errorcluster, "VISA resource name out"=w174:refnum<visa-resource-name>)  [unwired: 8 in]
        n76 = for {
          shift-right: [w190] -> w169
          shift-left: w173 -> [w186]
          shift-right: [w191] -> w170
          shift-left: w174 -> [w187]
          tunnel: w182 -> [w185] mode=indexing
          w184 = 0.0  # Voltage Level
          w188 = 0.0  # Current Limit
          w192 = T6 0 items=["Regulate", "Trip"] ("Behavior (0: Regulate)")
          n77 = Unbundle By Name(w185) -> ("Channel"=w189:T3)
          n78 = call "DP832_Configure Current Limit.vi"("Behavior"=w192, "error in (no error)"=w186, "Current Limit"=w188, "Channel"=w189, "VISA resource name"=w187) -> ("error out"=w194:errorcluster, "VISA resource name out"=w195:refnum<visa-resource-name>)  [unwired: 5 in]
          n79 = call "DP832_Configure Output.vi"("Enable Output (T: Enable)"=FALSE, "error in (no error)"=w194, "Voltage Level"=w184, "Channel"=w189, "VISA resource name"=w195) -> ("error out"=w190:errorcluster, "VISA resource name out"=w191:refnum<visa-resource-name>)  [unwired: 5 in]
        }
        n80 = call "DP832_Local Mode.vi"("error in (no error)"=w169, "VISA resource name"=w170) -> ("error out"=w172:errorcluster, "VISA resource name out"=w171:refnum<visa-resource-name>)  [unwired: 8 in]
        n81 = call "DP832_Close.vi"("error in (no error)"=w172, "VISA resource name"=w171) -> ("error out"=w168:errorcluster)  [unwired: 8 in, 1 out]
        n82 = Merge Errors(w168, w167, w166) -> (w177:errorcluster)
      }
      frame "Fin" {
        n83 = local read "Test"() -> (w197:bool)
        n84 = case shown="True" w197 {
          tunnel: w204 -> [_ w223]
          tunnel: w203 -> [_ w216]
          tunnel: w202 -> [_ w213]
          tunnel: w201 -> [_ w222]
          tunnel: w200 -> [w205 w217]
          tunnel: [w205 w218] -> w199
          frame False {
          }
          frame True {
            n85 = call "Reset.vi"("error in (no error)"=w217, "VISA resource name"=w216) -> ("error out"=w214:errorcluster, "VISA resource name out"=w215:refnum<visa-resource-name>)  [unwired: 8 out]
            n86 = call <instrlib>:"Close.vi"("error in (no error)"=w214, "VISA resource name"=w215) -> ("error out"=w219:errorcluster)  [unwired: 9 in]
            n87 = call "Reset.vi"("VISA resource name"=w213) -> ("error out"=w211:errorcluster, "VISA resource name out"=w212:refnum<visa-resource-name>)  [unwired: 9 in]
            n88 = call <instrlib>:"Close.vi"("error in (no error)"=w211, "VISA resource name"=w212) -> ("error out"=w220:errorcluster)  [unwired: 9 in]
            n89 = call "DP832_Enable ALL Output.vi"("Enable Output (T: Enable)"=FALSE, "VISA resource name"=w222) -> ("error out"=w226:errorcluster, "VISA resource name out"=w227:refnum<visa-resource-name>)  [unwired: 8 in]
            n90 = for {
              shift-right: [w235] -> w224
              shift-left: w226 -> [w231]
              shift-right: [w236] -> w225
              shift-left: w227 -> [w232]
              tunnel: w223 -> [w230] mode=indexing
              w229 = 0.0  # Voltage Level
              w233 = 0.0  # Current Limit
              w237 = T6 0 items=["Regulate", "Trip"] ("Behavior (0: Regulate)")
              n91 = Unbundle By Name(w230) -> ("Channel"=w234:T3)
              n92 = call "DP832_Configure Current Limit.vi"("Behavior"=w237, "error in (no error)"=w231, "Current Limit"=w233, "Channel"=w234, "VISA resource name"=w232) -> ("error out"=w239:errorcluster, "VISA resource name out"=w240:refnum<visa-resource-name>)  [unwired: 5 in]
              n93 = call "DP832_Configure Output.vi"("Enable Output (T: Enable)"=FALSE, "error in (no error)"=w239, "Voltage Level"=w229, "Channel"=w234, "VISA resource name"=w240) -> ("error out"=w235:errorcluster, "VISA resource name out"=w236:refnum<visa-resource-name>)  [unwired: 5 in]
            }
            n94 = local write "Test"(FALSE ("Test")) -> ()
            n95 = call "DP832_Local Mode.vi"("error in (no error)"=w224, "VISA resource name"=w225) -> ("error out"=w210:errorcluster, "VISA resource name out"=w209:refnum<visa-resource-name>)  [unwired: 8 in]
            n96 = call "Reset.vi"("error in (no error)"=w210, "VISA resource name"=w209) -> ("error out"=w207:errorcluster, "VISA resource name out"=w208:refnum<visa-resource-name>)  [unwired: 8 out]
            n97 = call "DP832_Close.vi"("error in (no error)"=w207, "VISA resource name"=w208) -> ("error out"=w221:errorcluster)  [unwired: 8 in, 1 out]
            n98 = Merge Errors(w221, w220, w219) -> (w218:errorcluster)
          }
        }
      }
      frame "Test Off" {
        w247 = FALSE
        n99 = local read "CONFIG GEN"() -> (w241:T1[])
        n100 = local read "VIn ASIC"() -> (w253:u16)
        n101 = Index Array(array=w241, index=w253) -> (element=w252:T1)
        n102 = Unbundle By Name(w252) -> ("Channel"=w251:u16, "Load"=w250:dbl)  [unwired: 11 out]
        n103 = call "Beep.vi"("VISA resource name"=w246, "error in (no error)"=w244, "Beep (T: ON)"=TRUE) -> ("VISA resource name out"=w245:refnum<visa-resource-name>, "error out"=w243:errorcluster)  [unwired: 11 in]
        n104 = call "Enable Output.vi"("VISA resource name"=w245, "Channel (1: Channel1)"=w251, "error in (no error)"=w243, "Enable Output (T: Enable)"=w247, "Enable Output Complement (T: Enable)"=w247, "Load (50 Ohm)"=w250) -> ("error out"=w249:errorcluster)  [unwired: 8 in, 1 out]
      }
      frame "Set default" {
        (unwired) T1 {"Channel"=1, "Frequency"=1000000.0, "Width Time"=3.3e-09, "Amplitude"=0.05, "DC Offset"=0.0, "Load"=500.0, "Leading Edge Time"=1e-09, "Trailing Edge Time"=1e-09, "Delay"=0.0, "Out"=TRUE, "/Out"=TRUE, "Trigger Level Sync"=1, "Trigger Sync Out"=1, "Vasic Theorical"=0.0} ("Config Pulse")
        n105 = One Button Dialog(message="Set values to default\n:)") -> ()  [unwired: 1 in, 1 out]
        n106 = call "gui.default values test.vi"() -> ("Values Generator"=w255:T1[])  [unwired: 7 in, 4 out]
        "Values Generator" <- w255
        n107 = local read "Test"() -> (w259:bool)
        n108 = Select(t=Machine_State_generador_pulsos."Test On" ("Enum"), s=w259, f=Machine_State_generador_pulsos."Idle" ("Enum")) -> (s? t:f=w256:T5)
        n109 = local write "CONFIG GEN"(w255) -> ()
      }
      frame "Cambio pulso" {
        n110 = local read "CONFIG GEN"() -> (w261:T1[])
        n111 = local read "Test"() -> (w265:bool)
        n112 = Select(t=Machine_State_generador_pulsos."Test On" ("Enum"), s=w265, f=Machine_State_generador_pulsos."Idle" ("Enum")) -> (s? t:f=w262:T5)
      }
      frame "Error Labview" {
        n113 = Unbundle By Name(w283) -> ("code"=w281:i32, "source"=w280:string)
        n114 = Format Into String(format string="Se ha producido un error interno.\nCodigo (%d).\n%s.", w281, w280) -> (resulting string=w276:string)  [unwired: 2 in, 1 out]
        n115 = call <vilib>:"Clear Errors.vi"("error in (no error)"=w283) -> ("error out"=w271:errorcluster)  [unwired: 5 in, 1 out]
        n116 = call <vilib>:"Three Button Dialog.vi"("Window Title (\"\")"="Error en labview" ("Window Title (\"\")"), "Right Button Text (\"Cancel\")"="Salir" ("Right Button Text (\"Cancel\")"), "Center Button Text (\"No\")"="Iniciar" ("Center Button Text (\"No\")"), "Left Button Text (\"Yes\")"="Reintentar" ("Left Button Text (\"Yes\")"), "message"=w276) -> ("Which Button?"=w274:T7)  [unwired: 6 in]
        n117 = case shown="\"Right Button\"" w274 {
          tunnel: w273 -> [w286 _ _]
          tunnel: [w286 Machine_State_generador_pulsos."Fin" ("y") Machine_State_generador_pulsos."Inicio" ("y")] -> w272
          tunnel: w271 -> [w285 w287 w297]
          tunnel: w270 -> [_ _ w296]
          tunnel: [w285 w287 w290] -> w269
          tunnel: w268 -> [_ _ w294]
          tunnel: w267 -> [_ _ w295]
          frame "Left Button", Default {
          }
          frame "Right Button" {
          }
          frame "Center Button" {
            n118 = call <instrlib>:"Close.vi"("VISA resource name"=w295) -> ("error out"=w292:errorcluster)  [unwired: 10 in]
            n119 = call <instrlib>:"Close.vi"("error in (no error)"=w297, "VISA resource name"=w296) -> ("error out"=w291:errorcluster)  [unwired: 9 in]
            n120 = call "DP832_Close.vi"("VISA resource name"=w294) -> ("error out"=w293:errorcluster)  [unwired: 9 in, 1 out]
            n121 = Merge Errors(w293, w292, w291) -> (w289:errorcluster)
            n122 = call <vilib>:"Clear Errors.vi"("error in (no error)"=w289) -> ("error out"=w290:errorcluster)  [unwired: 5 in, 1 out]
          }
        }
      }
      frame "Error maquina", Default {
        n123 = property on="Enum info" class="Enum (strict)"() -> ("Strings []"=w308:string[])  [unwired: 2 in, 2 out]
        n124 = Index Array(array=w308, index #1=w307, index #2=w306, index #3=w305) -> (element #1=w302:string, element #2=w301:string, element #3=w300:string)
        n125 = Format Into String(format string="\\n-%s\\n-%s\\n-%s\\n", initial string="Error en la maquina de estados!!!!\nUn estado no existe o no esta cableado,\nrevise el programa de labview para detectar\nese error.\nUltimos 3 estados:", w302, w301, w300) -> (resulting string=w299:string)  [unwired: 1 in, 1 out]
        n126 = Two Button Dialog(message=w299, 1:"Salir" ("F button name (\"Cancel\")"), 2:"Iniciar" ("T button name (\"OK\")")) -> (T button?=w312:bool)
        n127 = Select(t=Machine_State_generador_pulsos."Inicio" ("y"), s=w312, f=Machine_State_generador_pulsos."Fin" ("y")) -> (s? t:f=w309:T5)
      }
      frame "No salvar" {
        n128 = local read "CONFIG GEN origen"() -> (w317:T1[])
      }
    }
    n129 = Unbundle By Name(w24) -> ("status"=w21:bool)
    n130 = Equal?(x=w14, y=Machine_State_generador_pulsos."Bye") -> (x = y?=w23:bool)
    n131 = Compound Arithmetic op=OR(w23) -> (w22:bool)
    n132 = Select(t=Machine_State_generador_pulsos."Error Labview" ("y"), s=w21, f=w14) -> (s? t:f=w20:T5)
  }
  "error out" <- w9
  "Array pulse Out" <- w2
  n133 = disable-structure shown="Enabled" {
    frame Disabled {
      n134 = call <instrlib>:"Initialize.vi"() -> ("error out"=w324:errorcluster, "VISA resource name out"=w323:refnum<visa-resource-name>)  [unwired: 10 in]
      n135 = call <instrlib>:"VI Tree.vi"() -> ()  [unwired: 12 in]
      n136 = call <instrlib>:"Initialize.vi"("ID Query (True)"=FALSE) -> ("VISA resource name out"=w321:refnum<visa-resource-name>, "VISA resource name"=w320:refnum<visa-resource-name>)  [unwired: 8 in, 1 out]
      n137 = call <instrlib>:"Close.vi"("error in (no error)"=w324, "VISA resource name"=w323) -> ("error out"=w325:errorcluster)  [unwired: 9 in]
      n138 = call <instrlib>:"Close.vi"("VISA resource name"=w321) -> ()  [unwired: 10 in, 1 out]
      n139 = call <vilib>:"Clear Errors.vi"("error in (no error)"=w325) -> ()  [unwired: 5 in, 2 out]
      n140 = call <vilib>:"Clear Errors.vi"() -> ()  [unwired: 6 in, 2 out]
    }
    frame Enabled {
    }
  }
  n141 = disable-structure shown="Disabled" {
    disable-tunnel: w2 -> [w326 _]
    frame Disabled {
      n142 = flat-sequence {
        tunnel: w326 -> [_]
        frame #0 {
          n143 = control-ref of="This VI"() -> (w327:refnum<vi>)
          n144 = invoke class="VI" method="FP.Close"(reference=w327) -> ()  [unwired: 2 in, 3 out]
        }
      }
    }
    frame Enabled {
    }
  }
